vi "Example Get Array Pointer.vi"(8 "error in":errorcluster, 10 "PointerDatatype.lvclass":refnum<class "PointerDatatype.lvclass">, 11 "Array in":sgl[](array[numeric])=[3.0, 42.0, -21.3]) -> ()   [LabVIEW 2018]
uses:
  utils/PointerDatatype.lvclass
  Transcriptors/System API/Basic Datatypes Pointers/BooleanPointer.lvclass
  Transcriptors/System API/ArrayPointerFunction/ArrayFloat Get Pointer.vi
  Transcriptors/System API/BasicDatatypesPointerFunction/Float Get Pointer.vi
panel:
  out "x+y":u32
  out "error out":errorcluster
  out "element":refnum<class "BooleanPointer.lvclass">
  out "BooleanPointer.lvclass":refnum<class "BooleanPointer.lvclass">
  out "pointer":u32
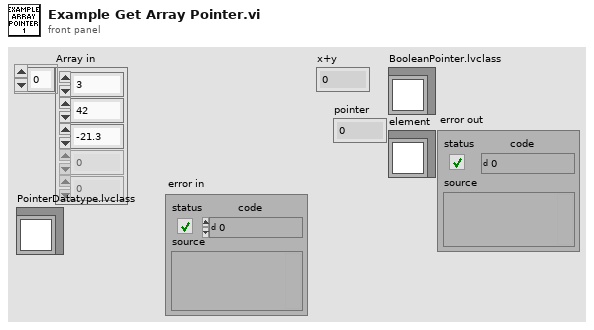
[diagram p1: front panel]
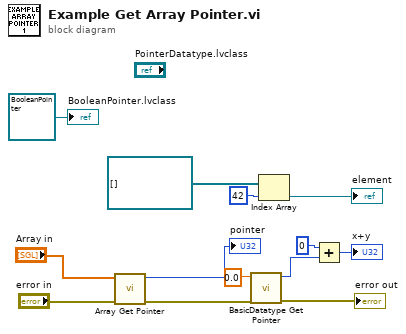
[diagram p0: block diagram]
diagram:
  n1 = call-poly "Array Get Pointer.vi"("error in"="error in", "float array in"="Array in") -> ("error out"=w1:errorcluster, "pointer"=→"pointer":u32)  [unwired: 8 in]
  n2 = call-poly "BasicDatatype Get Pointer.vi"("error in"=w1, "float in"=sgl 0.0) -> ("error out"=→"error out":errorcluster, "float pointer"=w4:u32)  [unwired: 8 in]
  n3 = Index Array(array=refnum<class "BooleanPointer.lvclass">[] [], index=42) -> (element=→"element":refnum<class "BooleanPointer.lvclass">)
  n4 = Add(x=u32 0, y=w4) -> (x+y=→"x+y":u32)
  "BooleanPointer.lvclass" <- refnum<class "BooleanPointer.lvclass"> refnum ("BooleanPointer.lvclass")
